vi "Refraction(subVI).vi"(8 "n2":dbl=1.333, 9 "n1":dbl=1.0, 10 "n":dbl[](array[numeric])=[0.0, 0.0, 1.0], 11 "v1":dbl[](array[numeric])=[1.0, 0.0, 1.0]) -> (3 "v2":dbl[](array[numeric])=[0.7501875468867217, 0.0, 1.1988405417302517])   [LabVIEW 2024]
uses:
  <vilib>/Analysis/_algsub.llb/Real Vector Norm.vi
  <vilib>/Analysis/baseanly.llb/Real Dot Product.vi
  <vilib>/Analysis/NI_AALBase.lvlib
  <vilib>/Analysis/NI_AALPro.lvlib
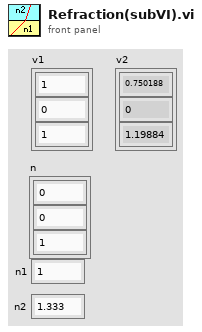
[diagram p1: front panel]
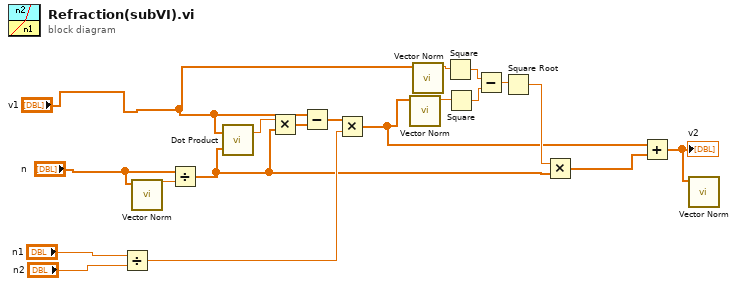
[diagram p0: block diagram]
diagram:
  n1 = Divide(x="n1", y="n2") -> (x/y=w14:dbl)
  n2 = call-poly <vilib>:"Vector Norm.vi"("Input Vector"="n") -> ("norm"=w12:dbl)  [unwired: 9 in, 1 out]
  n3 = Divide(x="n", y=w12) -> (x/y=w4:dbl[])
  n4 = call-poly <vilib>:"Dot Product.vi"("Y Vector"=w4, "X Vector"="v1") -> ("X * Y"=w19:dbl)  [unwired: 1 out]
  n5 = Multiply(x=w19, y=w4) -> (x*y=w18:dbl[])
  n6 = Subtract(x="v1", y=w18) -> (x-y=w17:dbl[])
  n7 = Multiply(x=w17, y=w14) -> (x*y=w2:dbl[])
  n8 = call-poly <vilib>:"Vector Norm.vi"("Input Vector"=w2) -> ("norm"=w9:dbl)  [unwired: 9 in, 1 out]
  n9 = call-poly <vilib>:"Vector Norm.vi"("Input Vector"="v1") -> ("norm"=w10:dbl)  [unwired: 9 in, 1 out]
  n10 = Square(x=w10) -> (x^2=w8:dbl)
  n11 = Square(x=w9) -> (x^2=w7:dbl)
  n12 = Subtract(x=w8, y=w7) -> (x-y=w6:dbl)
  n13 = Square Root(x=w6) -> (sqrt(x)=w5:dbl)
  n14 = Multiply(x=w5, y=w4) -> (x*y=w3:dbl[])
  n15 = Add(x=w2, y=w3) -> (x+y=w1:dbl[])
  "v2" <- w1
  n16 = call-poly <vilib>:"Vector Norm.vi"("Input Vector"=w1) -> ()  [unwired: 9 in, 2 out]
